vi "OpenSVObj.vi"(7 "AccessType":enum16{"Read", "Write"}(ring), 8 "error in":errorcluster, 11 "SVref":refnum<k21>) -> (0 "error out":errorcluster, 3 "SVref":refnum<k21>)   [LabVIEW 2016, in "Shared Variable Interface.lvlib" / "DBL.lvlib"]
uses:
  DBL.lvlib
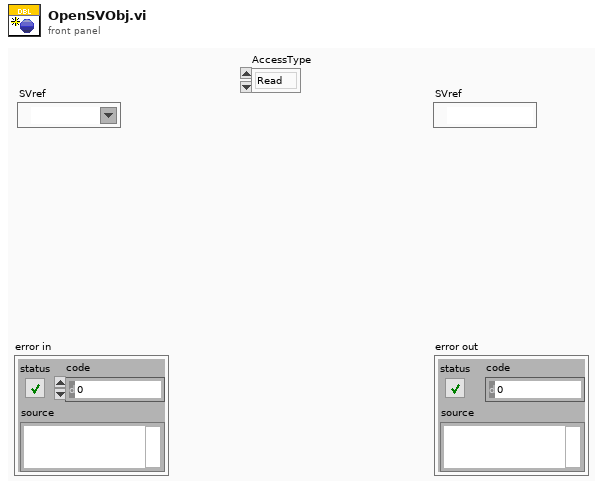
[diagram p1: front panel]
types:
  T1 = cluster{"Read Access":enum8{"Allowed", "Required", "None"}, "Write Access":enum8{"Allowed", "Required", "None"}}
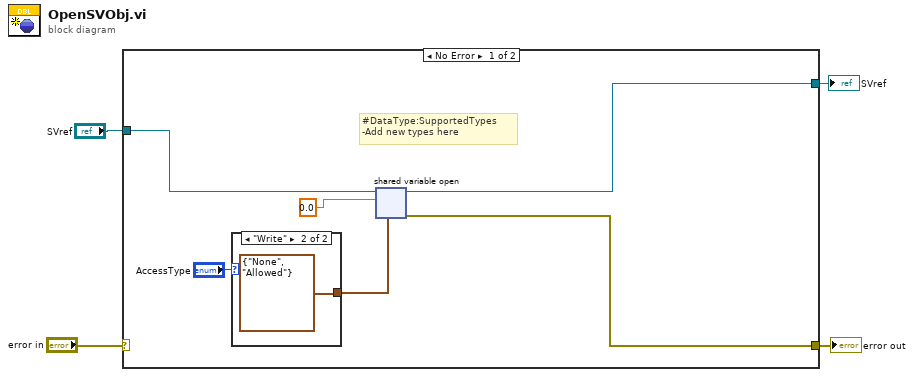
[diagram p0: block diagram]
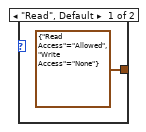
[diagram p2: hidden frame]
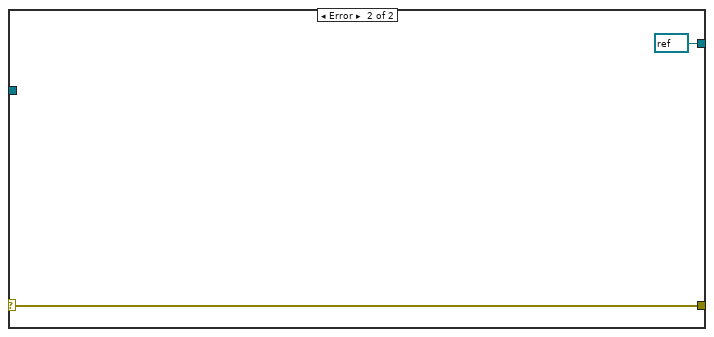
[diagram p3: hidden frame]
diagram:
  n1 = case shown="No Error" "error in" {
    selector: "error in" -> [_ w14]
    tunnel: [w9 w14] -> w4
    tunnel: "SVref" -> [w10 _]
    tunnel: [w5 refnum<k21> refnum ("SVref")] -> w1
    frame No Error {
      # "#DataType:SupportedTypes\n-Add new types here"
      n2 = case shown="\"Write\"" "AccessType" {
        tunnel: [T1 {"Read Access"=enum."Allowed", "Write Access"=enum."None"} ("access") T1 {"Read Access"=enum."None", "Write Access"=enum."Allowed"} ("access")] -> w7
        frame "Read", Default {
        }
        frame "Write" {
        }
      }
      n3 = shared-variable-open(w10, 0.0, w7) -> (w5:refnum<k21>, w9:errorcluster)  [unwired: 1 in]
    }
    frame Error {
    }
  }
  "error out" <- w4
  "SVref" <- w1
